vi "Simple TCP - Client.vi"() -> ()   [LabVIEW 2019]
doc: "演示连接TCP服务器、读取发送的数据并在图表上显示数据的方法。VI设计为TCP连接断开时停止。"
panel:
  in  "服务器关闭":string="服务器VI关闭了连接。"
  out "波形图":dbl[](graph)
  in  "停止":bool
  # "概述：演示使用TCP函数连接至TCP服务器VI并接收数据。\n操作步骤:\n1. 确保已运行Simple TCP - Server.vi。\n2.运行VI。\n3.单击停止按钮停止VI。注意，如停止服务器VI，该VI将自动停止。"
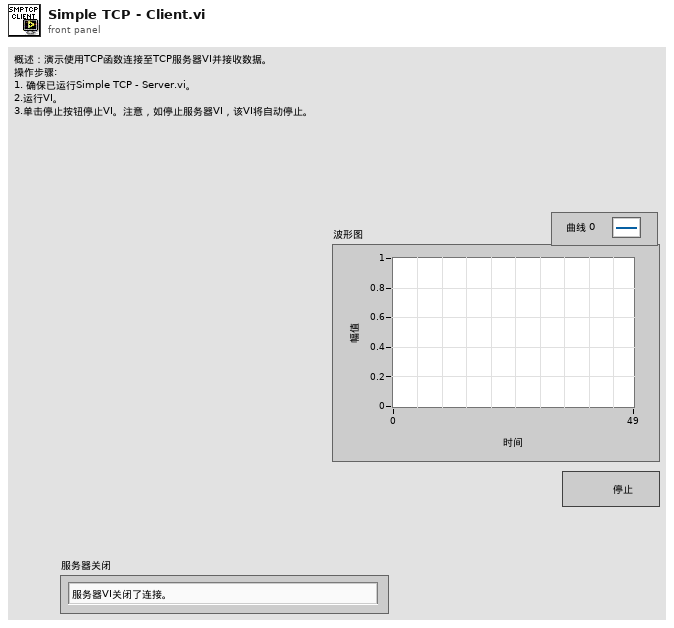
[diagram p1: front panel]
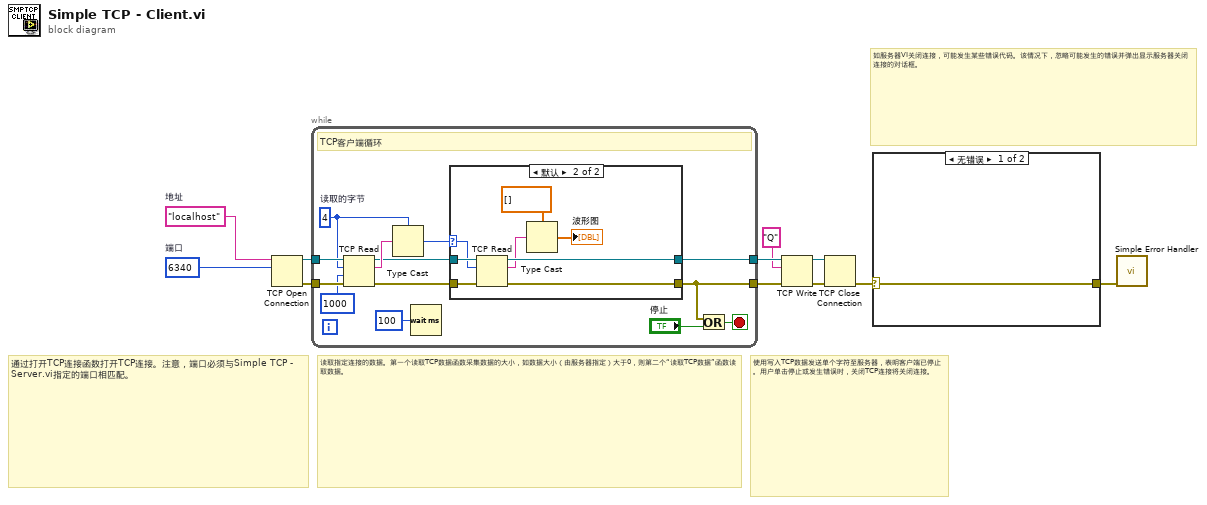
[diagram p0: block diagram]
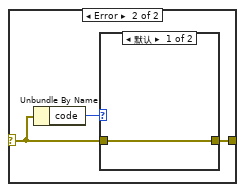
[diagram p2: hidden frame]
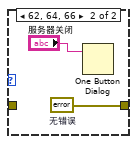
[diagram p3: hidden frame]
diagram:
  w1 = u16 6340  # 端口
  w2 = "localhost"  # 地址
  # "如服务器VI关闭连接，可能发生某些错误代码。该情况下，忽略可能发生的错误并弹出显示服务器关闭连接的对话框。"
  # "使用写入TCP数据发送单个字符至服务器，表明客户端已停止。用户单击停止或发生错误时，关闭TCP连接将关闭连接。"
  # "读取指定连接的数据。第一个读取TCP数据函数采集数据的大小，如数据大小（由服务器指定）大于0，则第二个“读取TCP数据”函数读取数据。"
  # "通过打开TCP连接函数打开TCP连接。注意，端口必须与Simple TCP - Server.vi指定的端口相匹配。"
  n1 = TCP Open Connection(address=w2, remote port or service name=w1) -> (connection ID=w11:refnum<k5>, error out=w10:errorcluster)  [unwired: 3 in]
  n2 = while {
    tunnel: w10 -> [w20]
    tunnel: w11 -> [w21]
    tunnel: [w15] -> w8
    tunnel: [w14] -> w6
    stop <- w17 stop-if-true
    w19 = 4  # 读取的字节
    # "TCP客户端循环"
    n3 = TCP Read(connection ID=w21, bytes to read=w19, error in (no error)=w20, 9:1000 ("timeout ms (25000)")) -> (connection ID out=w23:refnum<k5>, data out=w24:string, error out=w22:errorcluster)  [unwired: 1 in]
    n4 = Type Cast(type=w19, x=w24) -> (*(type *) &x=w13:i32)
    n5 = Wait (ms)(milliseconds to wait=u32 100) -> ()  [unwired: 1 out]
    n6 = case shown="默认" w13 {
      selector: w13 -> [_ w27]
      tunnel: w23 -> [w26 w34]
      tunnel: w22 -> [w25 w33]
      tunnel: [w26 w30] -> w15
      tunnel: [w25 w29] -> w14
      frame ..0 {
        # "服务器未写入任何数据"
      }
      frame Default {
        n7 = TCP Read(connection ID=w34, bytes to read=w27, error in (no error)=w33) -> (connection ID out=w30:refnum<k5>, data out=w28:string, error out=w29:errorcluster)  [unwired: 2 in]
        n8 = Type Cast(type=dbl[] [] ("chart"), x=w28) -> (*(type *) &x=→"波形图":dbl[])
      }
    }
    n9 = Or(x=w14, y="停止") -> (x .or. y?=w17:bool)
  }
  n10 = TCP Write(connection ID=w8, data in="Q", error in (no error)=w6) -> (connection ID out=w9:refnum<k5>, error out=w7:errorcluster)  [unwired: 2 out]
  n11 = TCP Close Connection(connection ID=w9, error in (no error)=w7) -> (error out=w4:errorcluster)  [unwired: 1 in, 1 out]
  n12 = case shown="无错误" w4 {
    selector: w4 -> [w35 w37]
    tunnel: [w35 w36] -> w3
    frame No Error {
    }
    frame Error {
      n13 = Unbundle By Name(w37) -> ("code"=w38:i32)
      n14 = case shown="默认" w38 {
        tunnel: w37 -> [w39 _]
        tunnel: [w39 w41] -> w36
        frame Default {
        }
        frame 62, 64, 66 {
          w41 = errorcluster {"status"=FALSE, "code"=0, "source"=""}  # 无错误
          n15 = One Button Dialog(message="服务器关闭") -> ()  [unwired: 1 in, 1 out]
        }
      }
    }
  }
  n16 = call <vilib>:"Simple Error Handler.vi"("error in (no error)"=w3) -> ()  [unwired: 4 in, 5 out]
